vi "FT_Set_Baud_Rate.vi"(8 "error in (no error)":errorcluster, 10 "Baud Rate":u32, 11 "Handle  In":u64) -> (0 "error out":errorcluster, 1 "FT_Status":u32(ring) items=["FT_OK", "FT_INVALID_HANDLE", "FT_DEVICE_NOT_FOUND", "FT_DEVICE_NOT_OPENED", "FT_IO_ERROR", "FT_INSUFFICIENT_RESOURCES", "FT_INVALID_PARAMETER", "FT_INVALID_BAUD_RATE", "FT_DEVICE_NOT_OPENED_FOR_ERASE", "FT_DEVICE_NOT_OPENED_FOR_WRITE", "FT_FAILED_TO_WRITE_DEVICE", "FT_EEPROM_READ_FAILED", "FT_EEPROM_WRITE_FAILED", "FT_EEPROM_ERASE_FAILED", "FT_EEPROM_NOT_PRESENT", "FT_EEPROM_NOT_PROGRAMMED", "FT_INVALID_ARGS", "FT_NOT_SUPPORTED", "FT_OTHER_ERROR"], 3 "Handle Out":u64)   [LabVIEW 2018]
uses:
  FTD2XX.dll
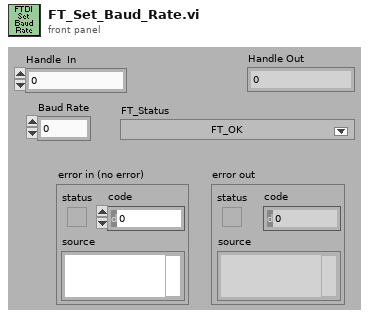
[diagram p1: front panel]
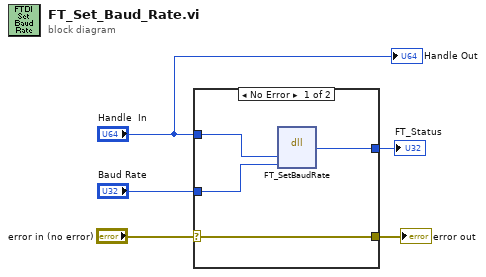
[diagram p0: block diagram]
diagram:
  n1 = case shown="No Error" "error in (no error)" {
    selector: "error in (no error)" -> [w6 w10]
    tunnel: [w9 _] -> w5
    tunnel: "Handle  In" -> [w8 _]
    tunnel: "Baud Rate" -> [w7 _]
    tunnel: [w6 w10] -> w1
    frame No Error {
      n2 = dll-call lib="FTD2XX.dll" fn="FT_SetBaudRate"("Handle"=w8, "BaudRate"=w7) -> ("FT_Status"=w9:u32)  [unwired: 5 in, 2 out]
    }
    frame Error {
    }
  }
  "FT_Status" <- w5
  "error out" <- w1
  "Handle Out" <- "Handle  In"
